vi "时间-光值曲线(子VI).vi"   [LabVIEW 2016, in "斯坦道CODMn.lvlib"]
uses:
  <vilib>/ptbypt/NI_PtbyPt.lvlib
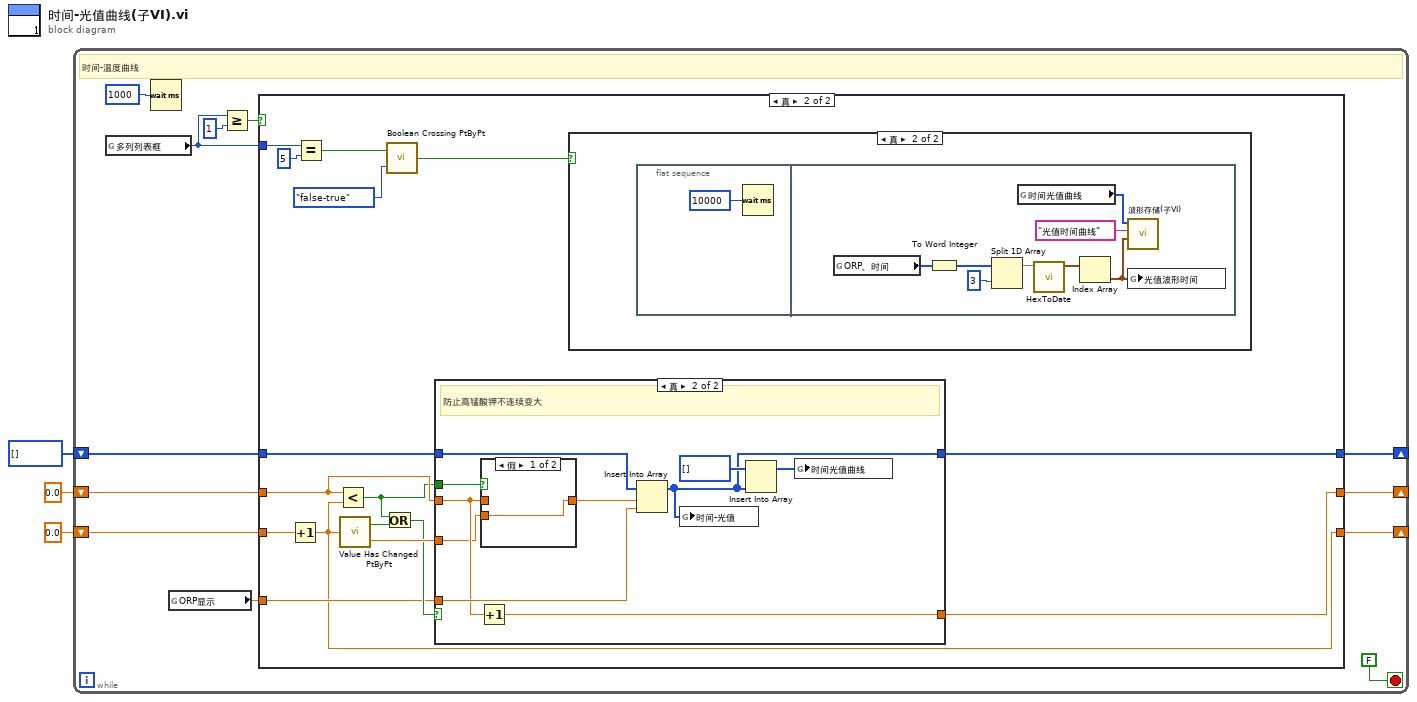
[diagram p0: block diagram]
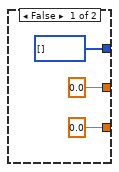
[diagram p2: hidden frame]
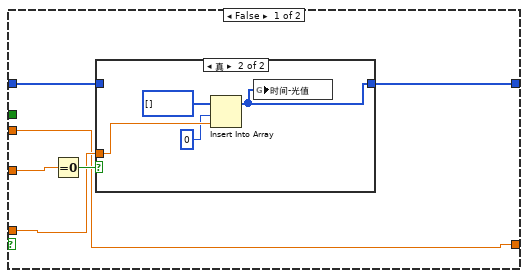
[diagram p4: hidden frame]
diagram:
  n1 = while {
    shift-right: [w12] -> _
    shift-left: u16[] [] ("ORP滴定曲线") -> [w13]
    shift-right: [w8] -> _
    shift-left: 0.0 -> [w9]
    shift-right: [w4] -> _
    shift-left: 0.0 -> [w6]
    stop <- FALSE stop-if-true
    # "时间-温度曲线"
    n2 = global read "运行时序全局变量.vi" "多列列表框"() -> (w7:i32)
    n3 = Wait (ms)(milliseconds to wait=u32 1000 ("等待时间（毫秒）")) -> ()  [unwired: 1 out]
    n4 = global read "COD内部交互全局.vi" "ORP显示"() -> (w5:dbl)
    n5 = Greater Or Equal?(x=w7, y=1) -> (x >= y?=w10:bool)
    n6 = case shown="真" w10 {
      tunnel: w13 -> [_ w34]
      tunnel: [u16[] [] ("ORP滴定曲线") w33] -> w12
      tunnel: w9 -> [_ w25]
      tunnel: [0.0 w24] -> w8
      tunnel: w7 -> [_ w22]
      tunnel: w6 -> [_ w21]
      tunnel: w5 -> [_ w20]
      tunnel: [0.0 w19] -> w4
      frame False {
      }
      frame True {
        n7 = Increment(x=w21) -> (x+1=w19:dbl)
        n8 = Equal?(x=w22, y=5) -> (x = y?=w29:bool)
        n9 = Less?(x=w25, y=w19) -> (x < y?=w23:bool)
        n10 = call <vilib>:"Value Has Changed PtByPt.vi"("input data point"=w19) -> ("has changed"=w32:bool, "output data point"=w31:dbl)  [unwired: 1 in]
        n11 = Or(x=w23, y=w32) -> (x .or. y?=w26:bool)
        n12 = call <vilib>:"Boolean Crossing PtByPt.vi"("direction"=enum16{"either", "false-true", "true-false"}."false-true", "input"=w29) -> ("crossing"=w27:bool)  [unwired: 1 in]
        n13 = case shown="真" w26 {
          tunnel: w34 -> [w48 w63]
          tunnel: [w47 w55] -> w33
          tunnel: w31 -> [w49 w57]
          tunnel: w20 -> [w45 w62]
          tunnel: w25 -> [w44 w59]
          tunnel: [w44 w61] -> w24
          tunnel: w23 -> [_ w60]
          frame False {
            n14 = Equal To 0?(x=w49) -> (x = 0?=w46:bool)
            n15 = case shown="真" w46 {
              tunnel: [w50 w51] -> w47
              tunnel: w48 -> [w50 _]
              tunnel: w45 -> [_ w53]
              frame False {
              }
              frame True {
                n16 = Insert Into Array(array=u16[] [] ("ORP滴定曲线"), index=0 ("索引"), new element=w53) -> (w51:u16[])
                n17 = global write "COD内部交互全局.vi" "时间-光值"(w51) -> ()
              }
            }
          }
          frame True {
            # "防止高锰酸钾不连续变大"
            n18 = Increment(x=w59) -> (x+1=w61:dbl)
            n19 = case shown="假" w60 {
              tunnel: w59 -> [_ w66]
              tunnel: [w65 w66] -> w58
              tunnel: w57 -> [w65 _]
              frame False {
              }
              frame True {
              }
            }
            n20 = Insert Into Array(array=w63, index=w58, new element=w62) -> (w55:u16[])
            n21 = global write "COD内部交互全局.vi" "时间-光值"(w55) -> ()
            n22 = Insert Into Array(array=u16[] [] ("ORP滴定曲线"), new element=w55) -> (w56:u16[])  [unwired: 1 in]
            n23 = global write "COD内部交互全局.vi" "时间光值曲线"(w56) -> ()
          }
        }
        n24 = case shown="真" w27 {
          frame False {
          }
          frame True {
            n25 = flat-sequence {
              frame #0 {
                n26 = Wait (ms)(milliseconds to wait=u32 10000 ("等待时间（毫秒）")) -> ()  [unwired: 1 out]
              }
              frame #1 {
                n27 = global read "COD内部交互全局.vi" "ORP、时间"() -> (w39:u16[])
                n28 = To Word Integer(number=w39) -> (16bit integer=w38:i16[])
                n29 = Split 1D Array(array=w38, index=3 ("索引")) -> (first subarray=w41:i16[])  [unwired: 1 out]
                n30 = global read "COD内部交互全局.vi" "时间光值曲线"() -> (w43:u16[])
                n31 = call "HexToDate.vi"("数组"=w41) -> ("DATE"=w40:timestamp[])  [unwired: 10 in]
                n32 = Index Array(array=w40) -> (element=w36:timestamp)  [unwired: 1 in]
                n33 = call "波形存储(子VI).vi"("波形时间"=w36, "condition"="光值时间曲线", "ORP滴定曲线"=w43) -> ()  [unwired: 9 in]
                n34 = global write "COD内部交互全局.vi" "光值波形时间"(w36) -> ()
              }
            }
          }
        }
      }
    }
  }
